vi "PRIME Detector Parse Status Message.vi"(8 "error in (no error)":errorcluster, 11 "JSON":string) -> (0 "error out":errorcluster, 3 "status":T1)   [LabVIEW 2021, in "PRIME Detector.lvclass"]
uses:
  PRIME Detector.lvclass
  PRIME Detector cluster Status.ctl
  294ab0f7-385b-46e2-99a9-bc3353a29e17.vi
  2235d8c1-8494-4036-afb4-fb3f392ebf9b.vi
  82dd99e6-2eb7-45f8-afd6-be02c65db71d.vi
  <vilib>/JDP Science/JSONtext/JSON text to Variant.vi
  <vilib>/JDP Science/JSONtext/LVClass Serializer/JSONtext LVClass Serializer.lvclass
  <vilib>/JDP Science/JSONtext/JSONtext.lvlib
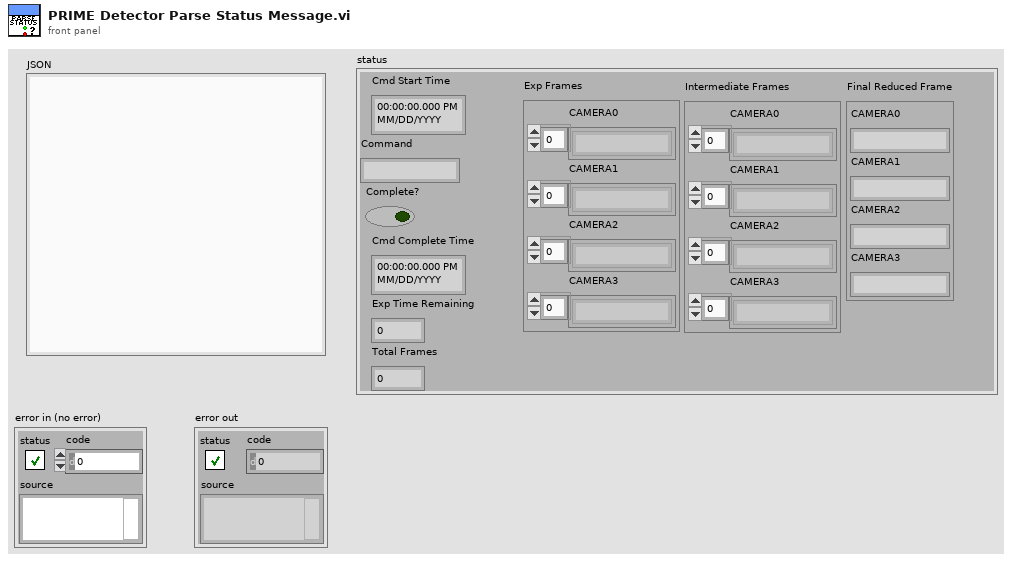
[diagram p1: front panel]
types:
  T1 = typedef "PRIME Detector cluster Status.ctl" = cluster{"Cmd Start Time":timestamp, "Command":string, "Complete?":bool, "Cmd Complete Time":timestamp, "Exp Time Remaining":dbl, "Total Frames":i32, "Exp Frames":cluster{"CAMERA0":string[], "CAMERA1":string[], "CAMERA2":string[], "CAMERA3":string[]}, "Intermediate Frames":cluster{"CAMERA0":string[], "CAMERA1":string[], "CAMERA2":string[], "CAMERA3":string[]}, "Final Reduced Frame":cluster{"CAMERA0":string, "CAMERA1":string, "CAMERA2":string, "CAMERA3":string}}
  T2 = cluster{"CAMERA0":string[], "CAMERA1":string[], "CAMERA2":string[], "CAMERA3":string[]}
  T3 = cluster{"CAMERA0":string, "CAMERA1":string, "CAMERA2":string, "CAMERA3":string}
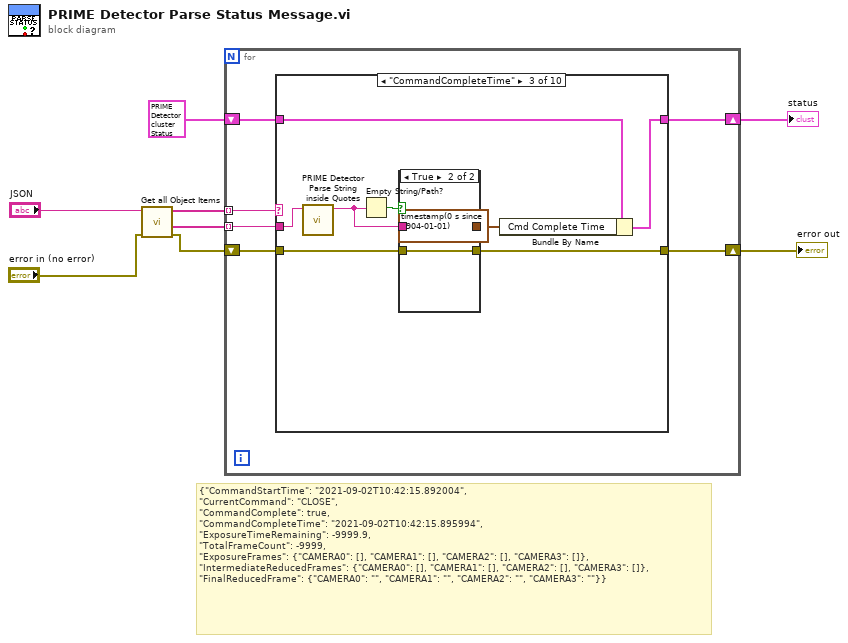
[diagram p0: block diagram]
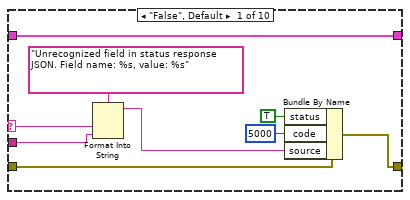
[diagram p2: hidden frame]
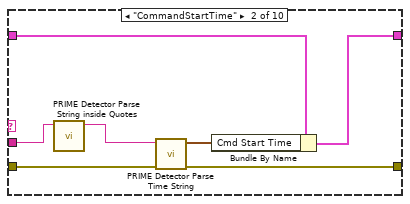
[diagram p3: hidden frame]
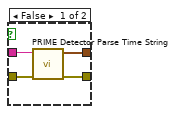
[diagram p4: hidden frame]
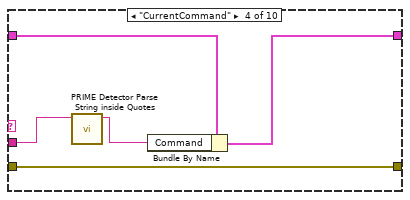
[diagram p5: hidden frame]
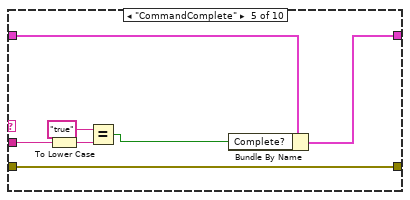
[diagram p6: hidden frame]
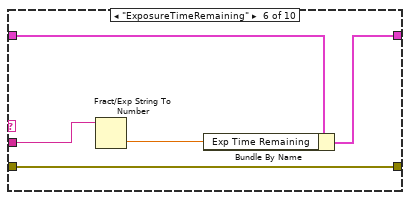
[diagram p7: hidden frame]
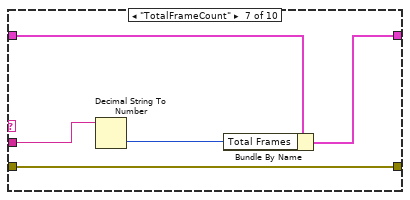
[diagram p8: hidden frame]
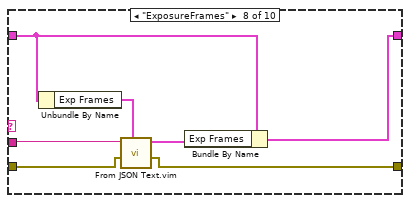
[diagram p9: hidden frame]
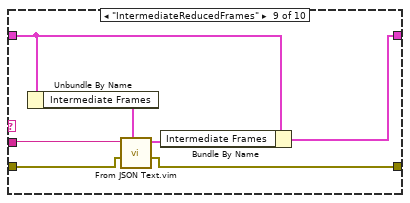
[diagram p10: hidden frame]
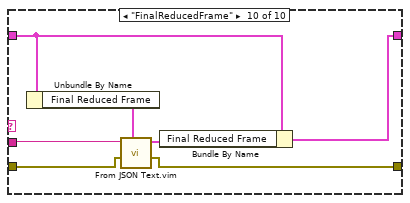
[diagram p11: hidden frame]
diagram:
  # "{\"CommandStartTime\": \"2021-09-02T10:42:15.892004\", \n\"CurrentCommand\": \"CLOSE\", \n\"CommandComplete\": true, \n\"CommandCompleteTime\": \"2021-09-02T10:42:15.895994\", \n\"ExposureTimeRemaining\": -9999.9, \n\"TotalFrameCount\": -9999, \n\"ExposureFrames\": {\"CAMERA0\": [], \"CAMERA1\": [], \"CAMERA2\": [], \"CAMERA3\": []}, \n\"IntermediateReducedFrames\": {\"CAMERA0\": [], \"CAMERA1\": [], \"CAMERA2\": [], \"CAMERA3\": []}, \n\"FinalReducedFrame\": {\"CAMERA0\": \"\", \"CAMERA1\": \"\", \"CAMERA2\": \"\", \"CAMERA3\": \"\"}}"
  n1 = call <vilib>:"Get all Object Items.vi"("error in (no error)"="error in (no error)", "JSON"="JSON") -> ("error out"=w3:errorcluster, "<JSON>"=w5:string[], "Item Names"=w6:string[])  [unwired: 6 in, 1 out]
  n2 = for {
    tunnel: w6 -> [w14] mode=indexing
    tunnel: w5 -> [w13] mode=indexing
    shift-right: [w10] -> w1
    shift-left: T1 {"Cmd Start Time"=timestamp(0 s since 1904-01-01), "Command"="", "Complete?"=FALSE, "Cmd Complete Time"=timestamp(0 s since 1904-01-01), "Exp Time Remaining"=0.0, "Total Frames"=0, "Exp Frames"={"CAMERA0"=[], "CAMERA1"=[], "CAMERA2"=[], "CAMERA3"=[]}, "Intermediate Frames"={"CAMERA0"=[], "CAMERA1"=[], "CAMERA2"=[], "CAMERA3"=[]}, "Final Reduced Frame"={"CAMERA0"="", "CAMERA1"="", "CAMERA2"="", "CAMERA3"=""}} -> [w11]
    shift-right: [w9] -> w2
    shift-left: w3 -> [w12]
    n3 = case shown="\"CommandCompleteTime\"" w14 {
      selector: w14 -> [w21 _ _ _ _ _ _ _ _ _]
      tunnel: w13 -> [w20 w24 w33 w46 w53 w58 w63 w72 w79 w86]
      tunnel: w12 -> [w19 w30 w38 w47 w54 w59 w64 w71 w78 w85]
      tunnel: w11 -> [w23 w29 w37 w49 w56 w61 w66 w70 w77 w84]
      tunnel: [w23 w27 w35 w48 w55 w60 w65 w68 w75 w82] -> w10
      tunnel: [w15 w26 w34 w47 w54 w59 w64 w67 w74 w81] -> w9
      frame "False", Default {
        n4 = Format Into String(format string="Unrecognized field in status response JSON. Field name: %s, value: %s", w21, w20) -> (resulting string=w18:string)  [unwired: 2 in, 1 out]
        n5 = Bundle By Name(cluster=w19, "status"=TRUE, "code"=5000, "source"=w18) -> (w15:errorcluster)
      }
      frame "CommandStartTime" {
        n6 = call "PRIME Detector Parse String inside Quotes.vi"("Quoted String"=w24) -> ("Contents of Quotes"=w25:string)  [unwired: 10 in]
        n7 = call "PRIME Detector Parse Time String.vi"("error in"=w30, "time string"=w25) -> ("error out"=w26:errorcluster, "time"=w28:timestamp)  [unwired: 8 in]
        n8 = Bundle By Name(cluster=w29, "Cmd Start Time"=w28) -> (w27:T1)
      }
      frame "CommandCompleteTime" {
        n9 = call "PRIME Detector Parse String inside Quotes.vi"("Quoted String"=w33) -> ("Contents of Quotes"=w32:string)  [unwired: 10 in]
        n10 = Empty String/Path?(string/path=w32) -> (empty?=w31:bool)
        n11 = case shown="True" w31 {
          tunnel: w38 -> [w42 w44]
          tunnel: [w41 timestamp(0 s since 1904-01-01) ("time")] -> w36
          tunnel: [w40 w44] -> w34
          tunnel: w32 -> [w39 _]
          frame False {
            n12 = call "PRIME Detector Parse Time String.vi"("error in"=w42, "time string"=w39) -> ("error out"=w40:errorcluster, "time"=w41:timestamp)  [unwired: 8 in]
          }
          frame True {
          }
        }
        n13 = Bundle By Name(cluster=w37, "Cmd Complete Time"=w36) -> (w35:T1)
      }
      frame "CurrentCommand" {
        n14 = call "PRIME Detector Parse String inside Quotes.vi"("Quoted String"=w46) -> ("Contents of Quotes"=w45:string)  [unwired: 10 in]
        n15 = Bundle By Name(cluster=w49, "Command"=w45) -> (w48:T1)
      }
      frame "CommandComplete" {
        n16 = To Lower Case(string=w53) -> (all lower case string=w52:string)
        n17 = Equal?(x="true", y=w52) -> (x = y?=w50:bool)
        n18 = Bundle By Name(cluster=w56, "Complete?"=w50) -> (w55:T1)
      }
      frame "ExposureTimeRemaining" {
        n19 = Fract/Exp String To Number(string=w58) -> (number=w57:dbl)  [unwired: 3 in, 1 out]
        n20 = Bundle By Name(cluster=w61, "Exp Time Remaining"=w57) -> (w60:T1)
      }
      frame "TotalFrameCount" {
        n21 = Decimal String To Number(string=w63) -> (number=w62:i32)  [unwired: 2 in, 1 out]
        n22 = Bundle By Name(cluster=w66, "Total Frames"=w62) -> (w65:T1)
      }
      frame "ExposureFrames" {
        n23 = Unbundle By Name(w70) -> ("Exp Frames"=w73:T2)
        n24 = call "From JSON Text.vim"("Data Type and Default Value"=w73, "error in (no error)"=w71, "JSON"=w72) -> ("error out"=w67:errorcluster, "Data out"=w69:T2)  [unwired: 7 in]
        n25 = Bundle By Name(cluster=w70, "Exp Frames"=w69) -> (w68:T1)
      }
      frame "IntermediateReducedFrames" {
        n26 = Unbundle By Name(w77) -> ("Intermediate Frames"=w80:T2)
        n27 = call "From JSON Text.vim"("Data Type and Default Value"=w80, "error in (no error)"=w78, "JSON"=w79) -> ("error out"=w74:errorcluster, "Data out"=w76:T2)  [unwired: 7 in]
        n28 = Bundle By Name(cluster=w77, "Intermediate Frames"=w76) -> (w75:T1)
      }
      frame "FinalReducedFrame" {
        n29 = Unbundle By Name(w84) -> ("Final Reduced Frame"=w87:T3)
        n30 = call "From JSON Text.vim"("Data Type and Default Value"=w87, "error in (no error)"=w85, "JSON"=w86) -> ("error out"=w81:errorcluster, "Data out"=w83:T3)  [unwired: 7 in]
        n31 = Bundle By Name(cluster=w84, "Final Reduced Frame"=w83) -> (w82:T1)
      }
    }
  }
  "status" <- w1
  "error out" <- w2
